vi "Main.vi"(10 "Nombre":string, 11 "Module Admin":refnum<class "Delacor_lib_QMH_Cloneable Module Admin.lvclass">) -> ()   [LabVIEW 2019, in "Inversor.lvlib"]
doc: "This template is based off of the Queued Message Handler design pattern and the Queued Message Handler project template that ships with LabVIEW.\n\nThe main difference is that the queue is private to this module and communication between modules is performed via Broadcast and Request events.\n\nRequest events are wrapped in public API methods and are handled in the Event Handling Loop (EHL) of this VI. Any module can register for Broadcast events sent by this module. The EHL generates messages based on user interface actions.\n\nThe Message Handling Loop (MHL) processes messages generated by the EHL, or by other messages. The messages are string values, so new messages can be added easily to the Message Cases case structure in the MHL. Each message cluster can also provide an optional value for Message Data, which is a variant that can be converted to whatever message-specific data is required.\n_____\nBased on DQMH Dev Tools: Project Template 7.1.0.1503."
uses:
  Inversor.lvlib
  <vilib>/Delacor/Delacor QMH/Libraries/Cloneable Module Admin_class/Delacor_lib_QMH_Cloneable Module Admin.lvclass
  C:/Program Files (x86)/National Instruments/LabVIEW 2024/vi.lib/Delacor/Delacor QMH/Libraries/Module Admin_class/Delacor_lib_QMH_Module Admin.lvclass
  Module Data--cluster.ctl
  <vilib>/Delacor/Delacor QMH/Libraries/Message Queue_class/Delacor_lib_QMH_Message Queue.lvclass/Delacor_lib_QMH_Message Queue.ctl
  <vilib>/Delacor/Delacor QMH/Libraries/Cloneable Module Admin_class/Delacor_lib_QMH_Cloneable Module Admin.lvclass/Delacor_lib_QMH_Cloneable Module Admin.ctl
  Stop Argument--cluster.ctl
  <vilib>/Delacor/Delacor QMH/Libraries/Module Admin_class/Delacor_lib_QMH_Module Admin.lvclass/Delacor_lib_QMH_Module Admin.ctl
  Request Privado Local Argument--cluster.ctl
  Request Privado Argument--cluster.ctl
  Set Voltage Argument--cluster.ctl
  Set Voltage (Reply Payload)--cluster.ctl
  Request Simple Argument--cluster.ctl
  <vilib>/Utility/miscctls.llb/LVPointTypeDef.ctl
  <vilib>/Delacor/Delacor QMH/Libraries/Message Queue_class/Delacor_lib_QMH_Enqueue Message (Single).vi
  <vilib>/Delacor/Delacor QMH/Libraries/Cloneable Module Admin_class/Delacor_lib_QMH_Get Module ID.vi
  <vilib>/Delacor/Delacor QMH/Libraries/Module Admin_class/Delacor_lib_QMH_Get External Launch.vi
  <vilib>/Delacor/Delacor QMH/Libraries/Message Queue_class/Delacor_lib_QMH_Message Queue.lvclass
panel:
  out "Active Modules (Array)":string[](array[string])
  in  "Select Module":i32(ring)=-1 caption="Select Module\nTo send Request to" items=["All"=-1]
  in  "Enviar Mensaje":bool
  in  "String":string
  out "error out":errorcluster
  out "Status":string
  in  "Simulate EHL Error":bool
  in  "Simulate MHL Error":bool
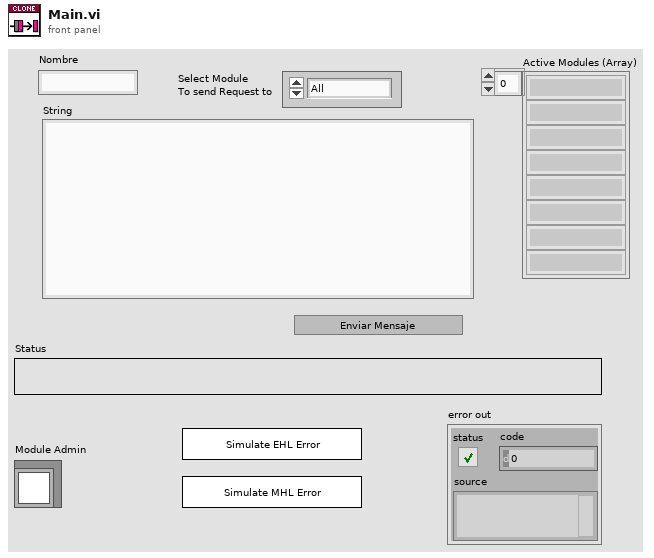
[diagram p1: front panel]
types:
  T1 = typedef "Inversor.lvlib/Broadcast Events--cluster.ctl" = cluster{"Module Did Init":refnum<user-event>, "Status Updated":refnum<user-event>, "Error Reported":refnum<user-event>, "Module Did Stop":refnum<user-event>, "Update Module Execution Status":refnum<user-event>}
  T2 = typedef "Inversor.lvlib/Request Events--cluster.ctl" = cluster{"Stop Module":refnum<user-event>, "Show Panel":refnum<user-event>, "Hide Panel":refnum<user-event>, "Show Diagram":refnum<user-event>, "Get Module Execution Status":refnum<user-event>, "Local Instance":T3, "Private.Request Privado":refnum<user-event>, "Set Voltage":refnum<user-event>, "Request Simple":refnum<user-event>}
  T3 = typedef "Inversor.lvlib/Local Instance Request Events--cluster.ctl" = cluster{"Request Privado Local":refnum<user-event>}
  T4 = typedef "Inversor.lvlib/Module Data--cluster.ctl" = cluster{"Status":string, "VISA resource name":refnum<visa-resource-name>}
  T5 = enum32{"invalid lock state", "Not Locked", "Locked (No Password)", "Password-protected"}
  T6 = typedef "Inversor.lvlib/Stop Argument--cluster.ctl" = cluster{"Module ID":i32, "Origin":string, "Exit via Stop Module Req?":bool, "Wait for Module to stop?":bool}
  T7 = typedef "Inversor.lvlib/Request Privado Local Argument--cluster.ctl" = cluster{"Module ID":i32, "Numeric":dbl}
  T8 = typedef "Inversor.lvlib/Request Privado Argument--cluster.ctl" = cluster{"Module ID":i32, "String":string}
  T9 = typedef "Inversor.lvlib/Set Voltage Argument--cluster.ctl" = cluster{"Module ID":i32, "Voltage":dbl, "Wait Notifier":refnum<notifier>, "wait for reply":bool}
  T10 = typedef "Inversor.lvlib/Request Simple Argument--cluster.ctl" = cluster{"Module ID":i32, "Numeric":dbl}
  T11 = typedef "LVPointTypeDef.ctl" = cluster{"Horizontal":i16, "Vertical":i16}
  T12 = enum32{"Invalid", "Standard", "Closed", "Hidden", "Minimized", "Maximized"}
  T13 = enum16{"Set Voltage", "Set Frecuency", "Set Speed", "Set Current"}
  T14 = typedef "Inversor.lvlib/Set Voltage (Reply Payload)--cluster.ctl" = cluster{"Module ID":i32, "Command":string, "error":errorcluster, "Response":string}
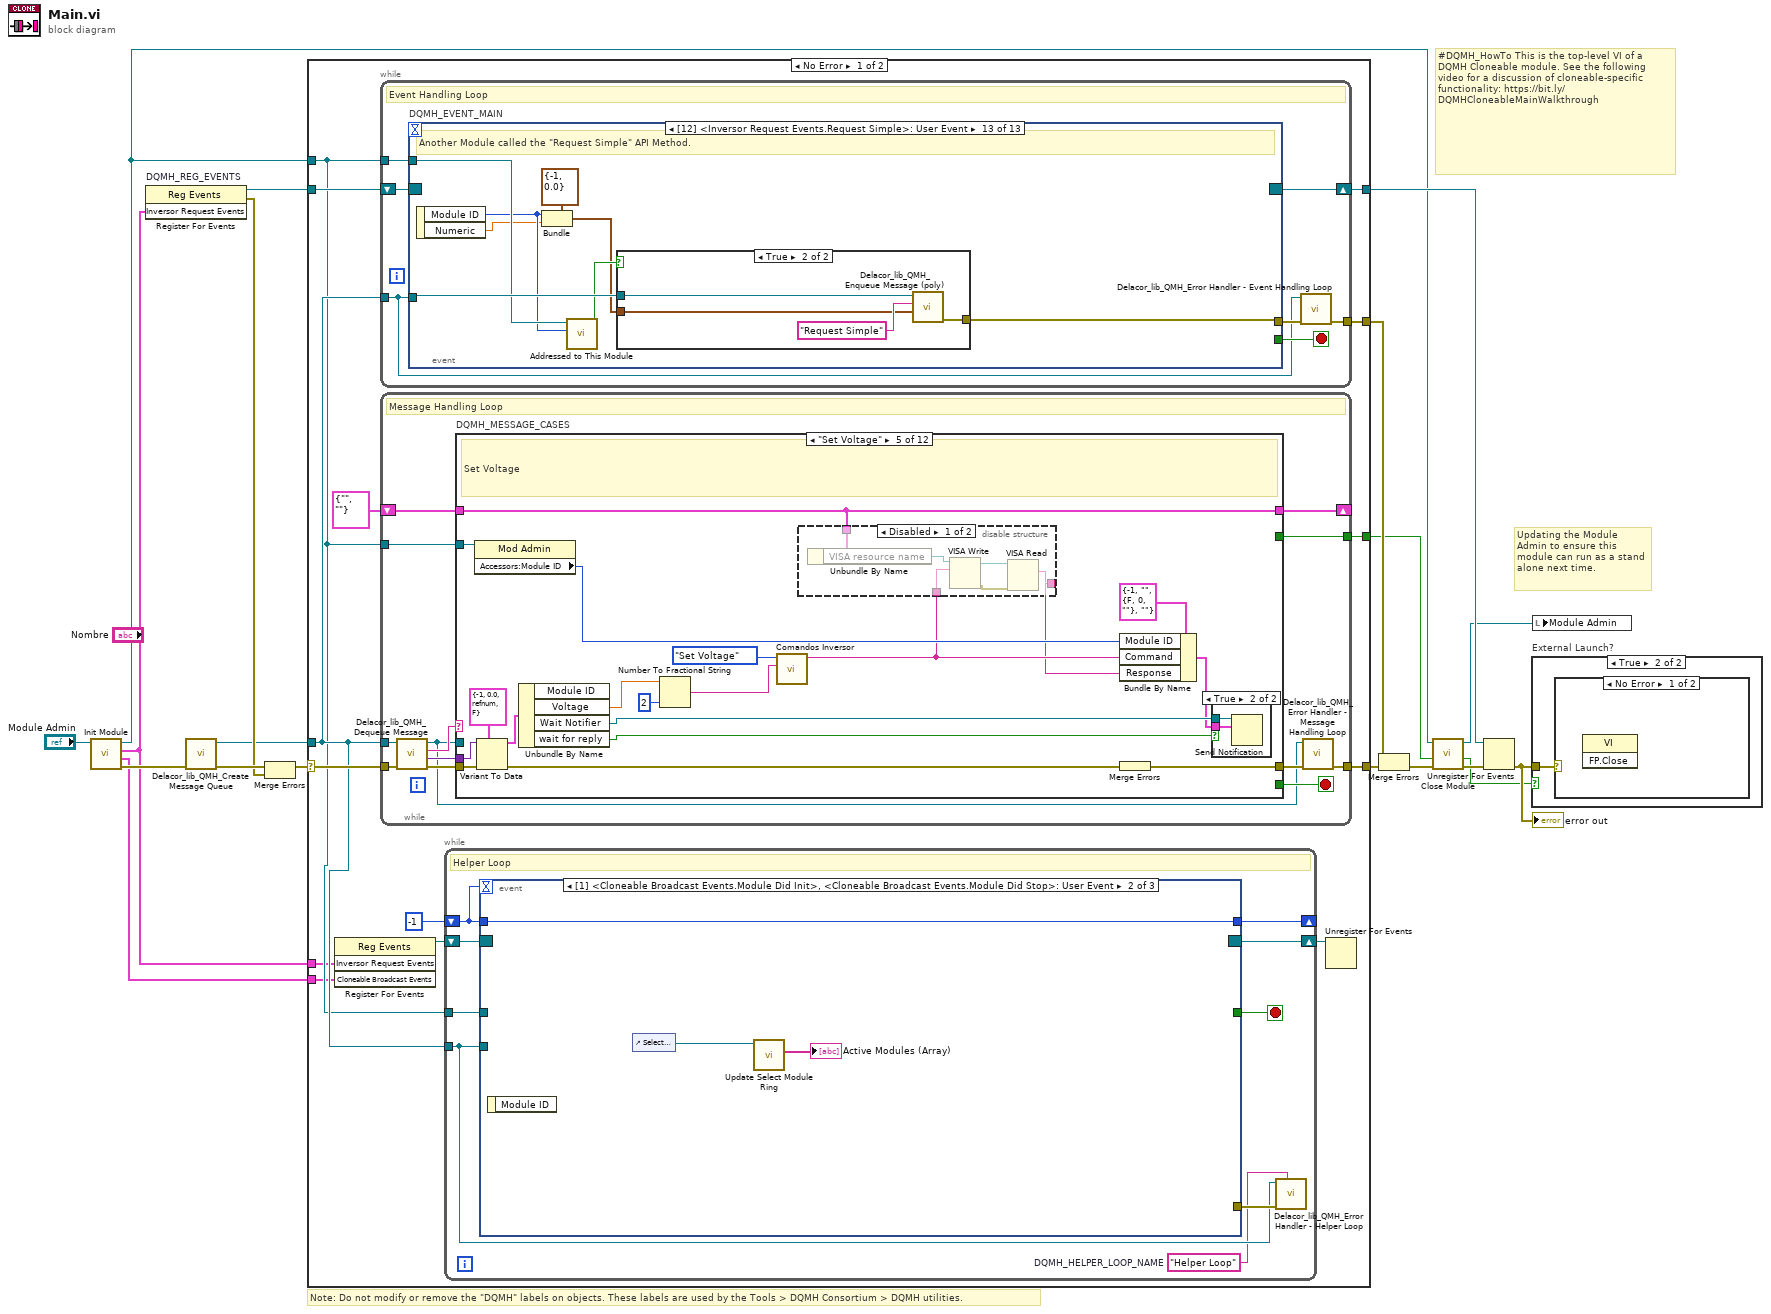
[diagram p0: block diagram]
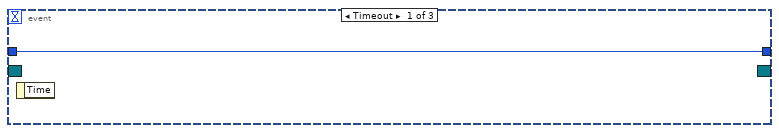
[diagram p2: hidden frame]
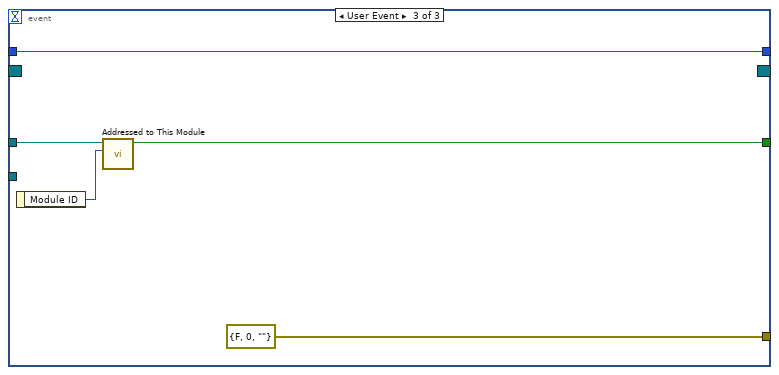
[diagram p3: hidden frame]
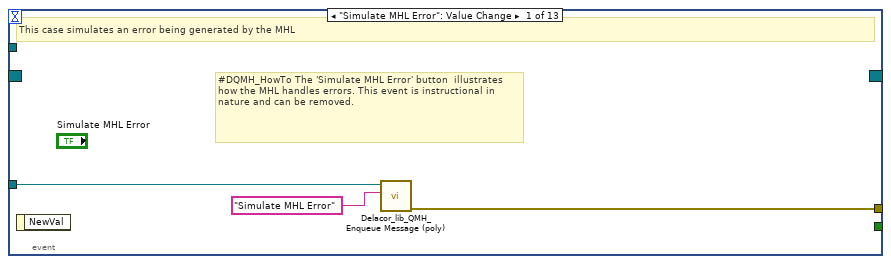
[diagram p4: hidden frame]
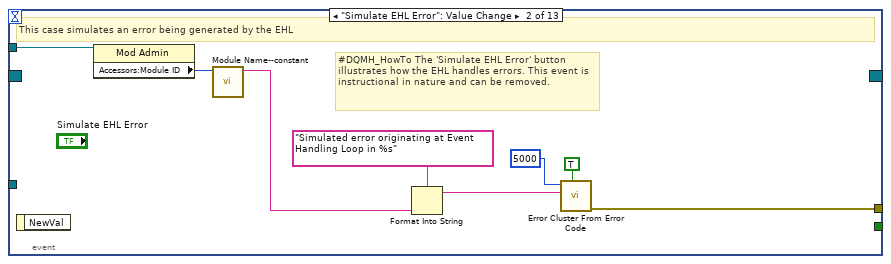
[diagram p5: hidden frame]
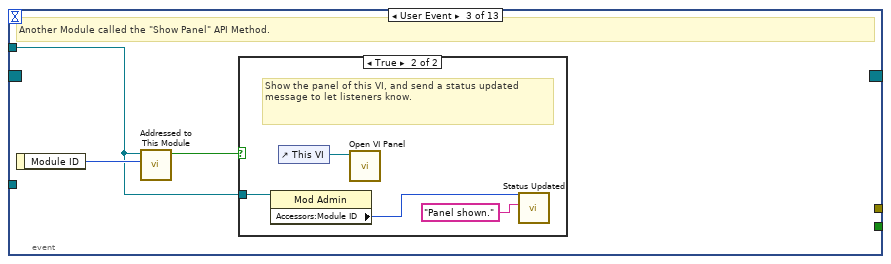
[diagram p6: hidden frame]
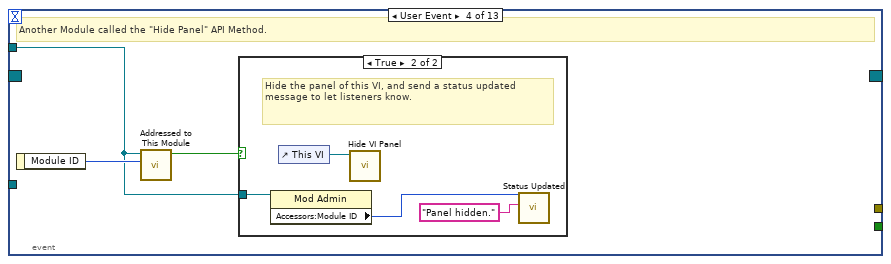
[diagram p8: hidden frame]
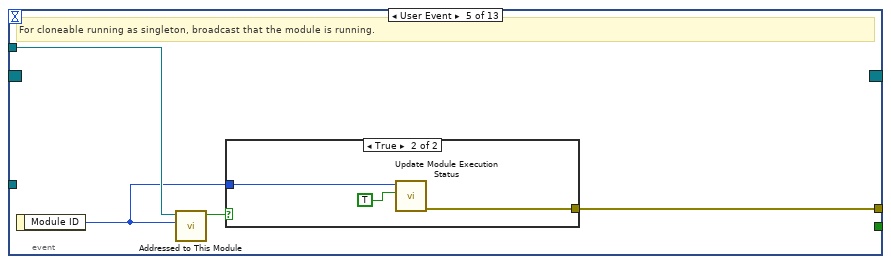
[diagram p10: hidden frame]
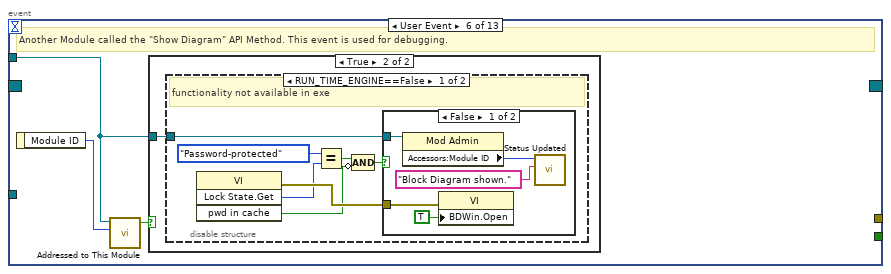
[diagram p12: hidden frame]
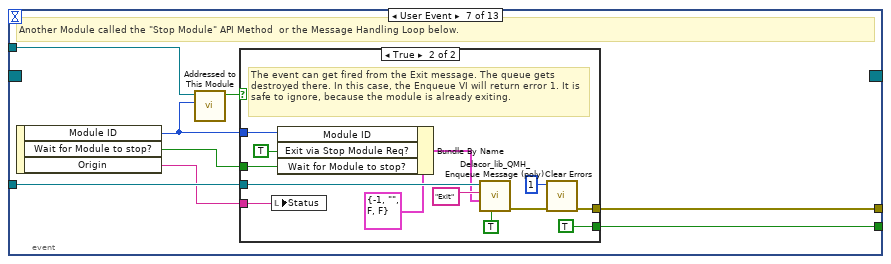
[diagram p16: hidden frame]
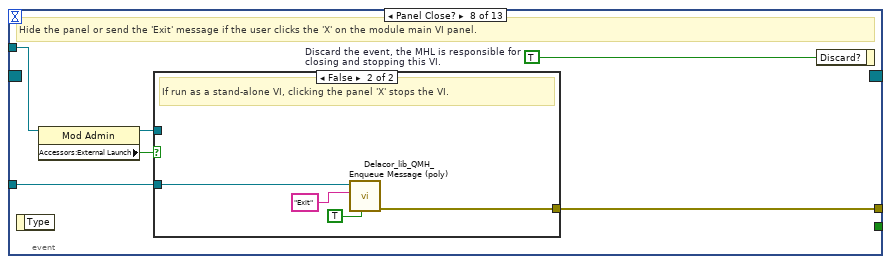
[diagram p18: hidden frame]
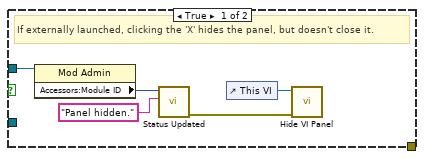
[diagram p19: hidden frame]
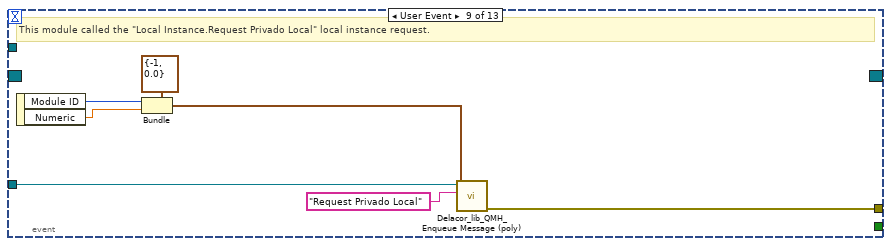
[diagram p20: hidden frame]
diagram:
  # "#DQMH_HowTo This is the top-level VI of a DQMH Cloneable module. See the following video for a discussion of cloneable-specific functionality: https://bit.ly/DQMHCloneableMainWalkthrough"
  # "Note: Do not modify or remove the \"DQMH\" labels on objects. These labels are used by the Tools > DQMH Consortium > DQMH utilities."
  # "Updating the Module Admin to ensure this module can run as a stand alone next time."
  n1 = call "Init Module.vi"("Cloneable Module Admin in"="Module Admin") -> ("error out"=w16:errorcluster, "Cloneable Broadcast Events"=w1:T1, "Inversor Request Events"=w2:T2, "Cloneable Module Admin out"=w6:refnum<class "Delacor_lib_QMH_Cloneable Module Admin.lvclass">)  [unwired: 7 in]
  n2 = register-events "DQMH_REG_EVENTS"(w2) -> (reference out=w9:refnum<event-registration>, error out=w11:errorcluster)  [unwired: 2 in]
  n3 = call <vilib>:"Delacor_lib_QMH_Create Message Queue.vi"("error in"=w16) -> ("error out"=w13:errorcluster, "Message Queue"=w8:refnum<class "Delacor_lib_QMH_Message Queue.lvclass">)  [unwired: 9 in]
  n4 = Merge Errors(w13, w11) -> (w12:errorcluster)
  n5 = case shown="No Error" w12 {
    selector: w12 -> [w31 w353]
    tunnel: [w33 w352] -> w17
    tunnel: [w30 w351] -> w10
    tunnel: w9 -> [w28 w351]
    tunnel: w8 -> [w27 w344]
    tunnel: [w32 _] -> w18
    tunnel: w6 -> [w26 w347]
    tunnel: [w25 _] -> w4
    tunnel: w2 -> [w24 _]
    tunnel: w1 -> [w20 _]
    frame No Error {
      n6 = register-events ("DQMH_HELPER_REGFOREVENTS")(w24, w20) -> (reference out=w22:refnum<event-registration>)  [unwired: 2 in, 1 out]
      n7 = while {
        tunnel: w27 -> [w52]
        shift-right: [w55] -> w30
        shift-left: w28 -> [w56]
        tunnel: [w57] -> w32
        tunnel: w26 -> [w53]
        stop <- w54 stop-if-true
        # "Event Handling Loop"
        n8 = event "DQMH_EVENT_MAIN" shown="[12] <Inversor Request Events.Request Simple>: User Event" {
          selector: w56 -> [_ _ _ _ _ _ _ _ _ _ _ _ _]
          dyn-events: [_ _ _ _ _ _ _ _ _ _ _ _ _] -> w55
          timeout: _ -> [_ _ _ _ _ _ _ _ _ _ _ _ _]
          tunnel: [_ _ _ _ _ _ w110 _ _ _ _ _ _] -> w54
          tunnel: w52 -> [w60 _ _ _ _ _ w113 w130 w149 w157 _ w173 w185]
          tunnel: [w61 w69 _ _ w87 _ w114 w133 w143 w150 _ w164 w178] -> w58
          tunnel: w53 -> [_ w68 w70 w77 w85 w91 w112 w131 _ w155 _ w171 w183]
          event "Simulate MHL Error": Value Change {
            # "#DQMH_HowTo The 'Simulate MHL Error' button  illustrates how the MHL handles errors. This event is instructional in nature and can be removed."
            # "This case simulates an error being generated by the MHL"
            n9 = event-data() -> ()  [unwired: 1 in, 1 out]
            n10 = call-poly <vilib>:"Delacor_lib_QMH_Enqueue Message (poly).vi"("Message"="Simulate MHL Error", "Message Queue in"=w60) -> ("error out"=w61:errorcluster)  [unwired: 8 in, 1 out]
          }
          event "Simulate EHL Error": Value Change {
            # "#DQMH_HowTo The 'Simulate EHL Error' button  illustrates how the EHL handles errors. This event is instructional in nature and can be removed."
            # "This case simulates an error being generated by the EHL"
            n11 = event-data() -> ()  [unwired: 1 in, 1 out]
            n12 = property on="Property Node" class="Mod Admin"(reference=w68) -> ("Accessors:Module ID"=w67:i32)  [unwired: 1 in, 2 out]
            n13 = call "Module Name--constant.vi"("Module ID"=w67) -> ("Module Name"=w62:string)  [unwired: 10 in]
            n14 = Format Into String(format string="Simulated error originating at Event Handling Loop in %s", w62) -> (resulting string=w65:string)  [unwired: 2 in, 1 out]
            n15 = call <vilib>:"Error Cluster From Error Code.vi"("show call chain? (False)"=TRUE, "error message (\"\")"=w65, "error code (0)"=5000) -> ("error out"=w69:errorcluster)  [unwired: 6 in]
          }
          event User Event {
            # "Another Module called the \"Show Panel\" API Method."
            n16 = event-data() -> ("Module ID"=w71:i32)  [unwired: 1 in]
            n17 = call "Addressed to This Module.vi"("Module ID from Argument"=w71, "Module Admin"=w70) -> ("Addressed to this instance?"=w72:bool)  [unwired: 8 in, 1 out]
            n18 = case shown="True" w72 {
              tunnel: w70 -> [_ w74]
              frame False {
              }
              frame True {
                # "Show the panel of this VI, and send a status updated message to let listeners know."
                n19 = property on="Property Node" class="Mod Admin"(reference=w74) -> ("Accessors:Module ID"=w73:i32)  [unwired: 1 in, 2 out]
                n20 = control-ref of="This VI"() -> (w76:refnum<vi>)
                n21 = call "Open VI Panel.vi"("VI"=w76) -> ()  [unwired: 10 in, 1 out]
                n22 = call "Status Updated.vi"("Status"="Panel shown." ("format string"), "Module ID"=w73) -> ()  [unwired: 9 in, 1 out]
              }
            }
          }
          event User Event {
            # "Another Module called the \"Hide Panel\" API Method."
            n23 = event-data() -> ("Module ID"=w78:i32)  [unwired: 1 in]
            n24 = call "Addressed to This Module.vi"("Module ID from Argument"=w78, "Module Admin"=w77) -> ("Addressed to this instance?"=w79:bool)  [unwired: 8 in, 1 out]
            n25 = case shown="True" w79 {
              tunnel: w77 -> [_ w81]
              frame False {
              }
              frame True {
                # "Hide the panel of this VI, and send a status updated message to let listeners know."
                n26 = property on="Property Node" class="Mod Admin"(reference=w81) -> ("Accessors:Module ID"=w80:i32)  [unwired: 1 in, 2 out]
                n27 = control-ref of="This VI"() -> (w83:refnum<vi>)
                n28 = call "Hide VI Panel.vi"("VI"=w83) -> ()  [unwired: 10 in, 1 out]
                n29 = call "Status Updated.vi"("Status"="Panel hidden." ("format string"), "Module ID"=w80) -> ()  [unwired: 9 in, 1 out]
              }
            }
          }
          event User Event {
            # "For cloneable running as singleton, broadcast that the module is running."
            n30 = event-data() -> ("Module ID"=w84:i32)  [unwired: 1 in]
            n31 = call "Addressed to This Module.vi"("Module ID from Argument"=w84, "Module Admin"=w85) -> ("Addressed to this instance?"=w86:bool)  [unwired: 8 in, 1 out]
            n32 = case shown="True" w86 {
              tunnel: [_ w90] -> w87
              tunnel: w84 -> [_ w89]
              frame False {
              }
              frame True {
                n33 = call "Update Module Execution Status.vi"("Running?"=TRUE, "Module ID"=w89) -> ("error out"=w90:errorcluster)  [unwired: 9 in]
              }
            }
          }
          event User Event {
            # "Another Module called the \"Show Diagram\" API Method. This event is used for debugging."
            n34 = event-data() -> ("Module ID"=w92:i32)  [unwired: 1 in]
            n35 = call "Addressed to This Module.vi"("Module ID from Argument"=w92, "Module Admin"=w91) -> ("Addressed to this instance?"=w93:bool)  [unwired: 8 in, 1 out]
            n36 = case shown="True" w93 {
              tunnel: w91 -> [_ w94]
              frame False {
              }
              frame True {
                n37 = disable-structure shown="RUN_TIME_ENGINE==False" {
                  disable-tunnel: w94 -> [w95 _]
                  frame condition #0 (active) {
                    # "functionality not available in exe"
                    n38 = invoke on="Invoke Node" class="VI" method="Lock State.Get"() -> (error out=w101:errorcluster, "Get Lock State"=w100:T5, "pwd in cache"=w97:bool)  [unwired: 4 in, 1 out]
                    n39 = Equal?(x=T5."Password-protected", y=w100) -> (x = y?=w98:bool)
                    n40 = Compound Arithmetic op=AND(w98, invert w97) -> (w96:bool)
                    n41 = case shown="False" w96 {
                      tunnel: w101 -> [w106 _]
                      tunnel: w95 -> [w103 _]
                      frame False {
                        n42 = property on="Property Node" class="Mod Admin"(reference=w103) -> ("Accessors:Module ID"=w102:i32)  [unwired: 1 in, 2 out]
                        n43 = property on="Property Node" class="VI"(error in=w106, "BDWin.Open"=TRUE ("Block Diagram Window:Open")) -> ()  [unwired: 1 in, 2 out]
                        n44 = call "Status Updated.vi"("Status"="Block Diagram shown." ("format string"), "Module ID"=w102) -> ()  [unwired: 9 in, 1 out]
                      }
                      frame True {
                        # "Password-protected VI, and the password is not in the cache. Do not show the diagram."
                      }
                    }
                  }
                  frame condition #1 {
                  }
                }
              }
            }
          }
          event User Event {
            # "Another Module called the \"Stop Module\" API Method  or the Message Handling Loop below."
            n45 = event-data() -> ("Module ID"=w108:i32, "Wait for Module to stop?"=w109:bool, "Origin"=w107:string)  [unwired: 1 in]
            n46 = call "Addressed to This Module.vi"("Module ID from Argument"=w108, "Module Admin"=w112) -> ("Addressed to this instance?"=w111:bool)  [unwired: 8 in, 1 out]
            n47 = case shown="True" w111 {
              tunnel: [_ w126] -> w114
              tunnel: w113 -> [_ w122]
              tunnel: [_ TRUE] -> w110
              tunnel: w109 -> [_ w117]
              tunnel: w108 -> [_ w119]
              tunnel: w107 -> [_ w115]
              frame False {
              }
              frame True {
                # "The event can get fired from the Exit message. The queue gets destroyed there. In this case, the Enqueue VI will return error 1. It is safe to ignore, because the module is already exiting."
                n48 = local write "Status"(w115) -> ()
                n49 = Bundle By Name(cluster=T6 {"Module ID"=-1, "Origin"="", "Exit via Stop Module Req?"=FALSE, "Wait for Module to stop?"=FALSE} ("Stop Argument"), "Module ID"=w119, "Exit via Stop Module Req?"=TRUE, "Wait for Module to stop?"=w117) -> (w116:T6)
                n50 = call-poly <vilib>:"Delacor_lib_QMH_Enqueue Message (poly).vi"("Priority Message? (F)"=TRUE, "Message Data"=w116, "Message"="Exit", "Message Queue in"=w122) -> ("error out"=w127:errorcluster)  [unwired: 6 in, 1 out]
                n51 = call <vilib>:"Clear Errors.vi"("error in (no error)"=w127, "specific error code to clear (0: all)"=1) -> ("error out"=w126:errorcluster)  [unwired: 4 in, 1 out]
              }
            }
          }
          event Panel Close? {
            w132 = TRUE  # Discard the event, the MHL is responsible for closing and stopping this VI.
            # "Hide the panel or send the 'Exit' message if the user clicks the 'X' on the module main VI panel."
            n52 = event-data() -> ()  [unwired: 1 in, 1 out]
            n53 = property on="Property Node" class="Mod Admin"(reference=w131) -> (reference out=w128:refnum<class "Delacor_lib_QMH_Cloneable Module Admin.lvclass">, "Accessors:External Launch"=w129:bool)  [unwired: 1 in, 1 out]
            n54 = case shown="False" w129 {
              tunnel: w130 -> [_ w141]
              tunnel: [_ w142] -> w133
              tunnel: w128 -> [w136 _]
              frame True {
                # "If externally launched, clicking the 'X' hides the panel, but doesn't close it."
                n55 = property on="Property Node" class="Mod Admin"(reference=w136) -> ("Accessors:Module ID"=w135:i32)  [unwired: 1 in, 2 out]
                n56 = call "Status Updated.vi"("Status"="Panel hidden." ("format string"), "Module ID"=w135) -> ("error out"=w134:errorcluster)  [unwired: 9 in]
                n57 = control-ref of="This VI"() -> (w138:refnum<vi>)
                n58 = call "Hide VI Panel.vi"("error in"=w134, "VI"=w138) -> ()  [unwired: 9 in, 1 out]
              }
              frame False {
                # "If run as a stand-alone VI, clicking the panel 'X' stops the VI."
                n59 = call-poly <vilib>:"Delacor_lib_QMH_Enqueue Message (poly).vi"("Priority Message? (F)"=TRUE, "Message"="Exit", "Message Queue in"=w141) -> ("error out"=w142:errorcluster)  [unwired: 7 in, 1 out]
              }
            }
            n60 = event-data ("Event Filter Node")("Discard?"=w132) -> ()  [unwired: 1 in, 1 out]
          }
          event User Event {
            # "This module called the \"Local Instance.Request Privado Local\" local instance request."
            n61 = event-data() -> ("Module ID"=w145:i32, "Numeric"=w144:dbl)  [unwired: 1 in]
            n62 = Bundle(cluster=T7 {"Module ID"=-1, "Numeric"=0.0} ("Request Privado Local Argument"), "Module ID"=w145, "Numeric"=w144) -> (w146:T7)
            n63 = call-poly <vilib>:"Delacor_lib_QMH_Enqueue Message (poly).vi"("Message Data"=w146, "Message"="Request Privado Local", "Message Queue in"=w149) -> ("error out"=w143:errorcluster)  [unwired: 7 in, 1 out]
          }
          event User Event {
            # "This module called the \"Private.Request Privado\" private request."
            n64 = event-data() -> ("Module ID"=w152:i32, "String"=w151:string)  [unwired: 1 in]
            n65 = Bundle(cluster=T8 {"Module ID"=-1, "String"=""} ("Request Privado Argument"), "Module ID"=w152, "String"=w151) -> (w153:T8)
            n66 = call "Addressed to This Module.vi"("Module ID from Argument"=w152, "Module Admin"=w155) -> ("Addressed to this instance?"=w156:bool)  [unwired: 8 in, 1 out]
            n67 = case shown="True" w156 {
              tunnel: w157 -> [_ w161]
              tunnel: w153 -> [_ w159]
              tunnel: [_ w158] -> w150
              frame False {
              }
              frame True {
                n68 = call-poly <vilib>:"Delacor_lib_QMH_Enqueue Message (poly).vi"("Message Data"=w159, "Message"="Request Privado", "Message Queue in"=w161) -> ("error out"=w158:errorcluster)  [unwired: 7 in, 1 out]
              }
            }
          }
          event "Enviar Mensaje": Value Change {
            n69 = event-data() -> ()  [unwired: 1 in, 1 out]
            n70 = call "Request Privado.vi"("String"="String", "Module ID"="Select Module") -> ()  [unwired: 9 in, 1 out]
          }
          event User Event {
            # "Another Module called the \"Set Voltage\" API Method."
            n71 = event-data() -> ("Module ID"=w168:i32, "Voltage"=w167:dbl, "Wait Notifier"=w166:refnum<notifier>, "wait for reply"=w165:bool)  [unwired: 1 in]
            n72 = Bundle(cluster=T9 {"Module ID"=-1, "Voltage"=0.0, "Wait Notifier"=refnum, "wait for reply"=FALSE} ("Set Voltage Argument"), "Module ID"=w168, "Voltage"=w167, "Wait Notifier"=w166, "wait for reply"=w165) -> (w169:T9)
            n73 = call "Addressed to This Module.vi"("Module ID from Argument"=w168, "Module Admin"=w171) -> ("Addressed to this instance?"=w172:bool)  [unwired: 8 in, 1 out]
            n74 = case shown="True" w172 {
              tunnel: w173 -> [_ w177]
              tunnel: w169 -> [_ w175]
              tunnel: [_ w174] -> w164
              frame False {
              }
              frame True {
                n75 = call-poly <vilib>:"Delacor_lib_QMH_Enqueue Message (poly).vi"("Message Data"=w175, "Message"="Set Voltage", "Message Queue in"=w177) -> ("error out"=w174:errorcluster)  [unwired: 7 in, 1 out]
              }
            }
          }
          event User Event {
            # "Another Module called the \"Request Simple\" API Method."
            n76 = event-data() -> ("Module ID"=w180:i32, "Numeric"=w179:dbl)  [unwired: 1 in]
            n77 = Bundle(cluster=T10 {"Module ID"=-1, "Numeric"=0.0} ("Request Simple Argument"), "Module ID"=w180, "Numeric"=w179) -> (w181:T10)
            n78 = call "Addressed to This Module.vi"("Module ID from Argument"=w180, "Module Admin"=w183) -> ("Addressed to this instance?"=w184:bool)  [unwired: 8 in, 1 out]
            n79 = case shown="True" w184 {
              tunnel: w185 -> [_ w189]
              tunnel: w181 -> [_ w187]
              tunnel: [_ w186] -> w178
              frame False {
              }
              frame True {
                n80 = call-poly <vilib>:"Delacor_lib_QMH_Enqueue Message (poly).vi"("Message Data"=w187, "Message"="Request Simple", "Message Queue in"=w189) -> ("error out"=w186:errorcluster)  [unwired: 7 in, 1 out]
              }
            }
          }
        }
        n81 = call-dynamic "Delacor_lib_QMH_Error Handler - Event Handling Loop.vi"("error in"=w58, "Message Queue in"=w52) -> ("dup error in"=w57:errorcluster)  [unwired: 8 in, 1 out]
      }
      n82 = while {
        tunnel: w27 -> [w190]
        shift-right: [w197] -> _
        shift-left: T4 {"Status"="", "VISA resource name"=""} ("Data Cluster") -> [w198]
        tunnel: w31 -> [w201]
        tunnel: [w199] -> w33
        tunnel: w26 -> [w192]
        tunnel: [w191] -> w25
        stop <- w196 stop-if-true
        # "Message Handling Loop"
        n83 = call-dynamic "Delacor_lib_QMH_Dequeue Message.vi"("error in"=w201, "Message Queue in"=w190) -> ("error out"=w200:errorcluster, "Message Data"=w194:variant, "Message"=w195:string, "Message Queue out"=w193:refnum<class "Delacor_lib_QMH_Message Queue.lvclass">)  [unwired: 6 in]
        n84 = case "DQMH_MESSAGE_CASES" shown="\"Set Voltage\"" w195 {
          selector: w195 -> [_ _ _ _ _ _ _ _ _ _ _ w333]
          tunnel: w193 -> [_ _ _ _ _ _ _ _ w288 _ w325 _]
          tunnel: w200 -> [w222 w226 w232 w243 w262 w280 w283 w285 w297 w314 w331 w342]
          tunnel: [w220 w226 w230 w241 w253 w278 w282 w285 w293 w313 w326 w343] -> w202
          tunnel: w198 -> [w213 w225 w231 w242 w246 w279 w281 w284 w292 w311 w324 w340]
          tunnel: [w212 w225 w231 w242 w246 w279 w281 w284 w292 w311 w324 w340] -> w197
          tunnel: [_ _ _ _ _ _ _ _ _ _ w323 _] -> w196
          tunnel: w194 -> [_ _ w229 w240 w260 w277 _ _ w291 _ w321 _]
          tunnel: w192 -> [w208 _ _ w237 w251 w274 _ _ w290 w309 w316 w339]
          tunnel: [_ _ _ _ _ _ _ _ _ _ w319 _] -> w191
          frame "Initialize" {
            w205 = "Initial Message" ("Initial Message")
            # "#DQMH_CodeNeeded - Initialize the appearance of the front panel."
            # "#DQMH_CodeNeeded - Initialize your state data here."
            # "Initialize - Any operation that needs to be done before the module can receive messages. Synchronize Caller Events.vi will inform Start Module.vi that the module has launched and is ready to receive messages. Module Did Init.vi will broadcast that the module initialized."
            n85 = call "Synchronize Caller Events.vi"("error in"=w222, "Module Admin"=w208) -> ("error out"=w221:errorcluster, "Module Admin out"=w207:refnum<class "Delacor_lib_QMH_Cloneable Module Admin.lvclass">)  [unwired: 8 in]
            n86 = property on="Property Node" class="Mod Admin"(reference=w207) -> ("Accessors:Module ID"=w204:i32, "Accessors:External Launch"=w209:bool)  [unwired: 1 in, 2 out]
            n87 = call "Module Name--constant.vi"("Module ID"=w204) -> ("Module Name"=w217:string)  [unwired: 10 in]
            n88 = property on="Property Node" class="VI"("Front Panel.Title"=w217) -> (reference out=w219:refnum<vi>, error out=w224:errorcluster)  [unwired: 2 in]
            n89 = Select(t=T12."Hidden" ("State"), s=w209, f=T12."Standard" ("State")) -> (s? t:f=w214:T12)
            n90 = invoke on="Invoke Node" class="VI" method="FP.Open"(reference=w219, error in=w224, "State"=w214) -> (reference out=w218:refnum<vi>, error out=w223:errorcluster)  [unwired: 2 in, 3 out]
            n91 = Bundle By Name(cluster=w213, "Status"=w205) -> (w212:T4)
            n92 = invoke on="Invoke Node" class="VI" method="FP.Center"(reference=w218, error in=w223) -> ()  [unwired: 1 in, 3 out]
            n93 = property on="Pane" class="Pane"("Origin"=T11 {"Horizontal"=0, "Vertical"=0}) -> ()  [unwired: 2 in, 2 out]
            n94 = call "Request Privado Local.vi"("Numeric"=123.0, "Module ID"=w204) -> ()  [unwired: 9 in, 1 out]
            n95 = call "Module Name--constant.vi"("Module ID"=w204) -> ("Module Name"=w210:string)  [unwired: 10 in]
            n96 = call "Module Did Init.vi"("error in"=w221, "Initialized?"=TRUE, "Origin"=w210, "Module ID"=w204) -> ("error out"=w220:errorcluster)  [unwired: 7 in]
            "Status" <- w205
          }
          frame "---Module Specific---" {
            # "Separator -- The following cases handle messages specific to this Module."
          }
          frame "Request Privado Local" {
            n97 = Variant To Data(error in=w232, type=T7 {"Module ID"=-1, "Numeric"=0.0} ("Request Privado Local Argument"), Variant=w229) -> (data=w227:T7, error out=w230:errorcluster)
            n98 = Unbundle By Name(w227) -> ()  [unwired: 2 out]
          }
          frame "Request Privado" {
            n99 = Variant To Data(error in=w243, type=T8 {"Module ID"=-1, "String"=""} ("Request Privado Argument"), Variant=w240) -> (data=w238:T8, error out=w241:errorcluster)
            n100 = property class="Mod Admin"(reference=w237) -> ("Accessors:Module ID"=w236:i32)  [unwired: 1 in, 2 out]
            n101 = Unbundle By Name(w238) -> ("String"=w235:string)
            n102 = Format Into String(format string="Module ID:%d Mensaje recibido: %s", w236, w235) -> (resulting string=w234:string)  [unwired: 2 in, 1 out]
            n103 = One Button Dialog(message=w234) -> ()  [unwired: 1 in, 1 out]
          }
          frame "Set Voltage" {
            # "Set Voltage"
            n104 = property class="Mod Admin"(reference=w251) -> ("Accessors:Module ID"=w252:i32)  [unwired: 1 in, 2 out]
            n105 = Variant To Data(error in=w262, type=T9 {"Module ID"=-1, "Voltage"=0.0, "Wait Notifier"=refnum, "wait for reply"=FALSE} ("Set Voltage Argument"), Variant=w260) -> (data=w258:T9, error out=w261:errorcluster)
            n106 = Unbundle By Name(w258) -> ("Voltage"=w249:dbl, "Wait Notifier"=w257:refnum<notifier>, "wait for reply"=w256:bool)  [unwired: 1 out]
            n107 = Number To Fractional String(number=w249, precision (6)=i16 2) -> (F-format string=w248:string)  [unwired: 2 in]
            n108 = call "Comandos Inversor.vi"("Argument"=w248, "Command"=T13."Set Voltage") -> ("Command"=w245:string)  [unwired: 9 in]
            n109 = disable-structure shown="Disabled" {
              disable-tunnel: w246 -> [w268 _]
              disable-tunnel: w245 -> [w266 _]
              disable-tunnel: [w263 _] -> w244
              frame Disabled {
                n110 = Unbundle By Name(w268) -> ("VISA resource name"=w267:refnum<visa-resource-name>)
                n111 = VISA Write(VISA resource name=w267, write buffer=w266) -> (VISA resource name out=w265:refnum<visa-resource-name>, error out=w264:errorcluster)  [unwired: 1 in, 1 out]
                n112 = VISA Read(VISA resource name=w265, error in (no error)=w264) -> (read buffer=w263:string)  [unwired: 1 in, 3 out]
              }
              frame Enabled {
              }
            }
            n113 = Bundle By Name(cluster=T14 {"Module ID"=-1, "Command"="", "error"={"status"=FALSE, "code"=0, "source"=""}, "Response"=""} ("Set Voltage (Reply Payload)"), "Module ID"=w252, "Command"=w245, "Response"=w244) -> (w255:T14)
            n114 = Merge Errors(w261) -> (w253:errorcluster)
            n115 = case "DQMH_FIRE_NOTIFIER" shown="True" w256 {
              tunnel: w257 -> [_ w270]
              tunnel: w255 -> [_ w269]
              frame False {
              }
              frame True {
                n116 = Send Notification(notification=w269, notifier=w270) -> ()  [unwired: 1 in, 2 out]
              }
            }
          }
          frame "Request Simple" {
            n117 = Variant To Data(error in=w280, type=T10 {"Module ID"=-1, "Numeric"=0.0} ("Request Simple Argument"), Variant=w277) -> (data=w275:T10, error out=w278:errorcluster)
            n118 = Unbundle By Name(w275) -> ("Numeric"=w272:dbl)  [unwired: 1 out]
            n119 = property class="Mod Admin"(reference=w274) -> ("Accessors:Module ID"=w273:i32)  [unwired: 1 in, 2 out]
            n120 = Format Into String(w272) -> (resulting string=w271:string)  [unwired: 3 in, 1 out]
            n121 = call "Status Updated.vi"("Status"=w271, "Module ID"=w273) -> ()  [unwired: 9 in, 1 out]
          }
          frame "---Copy This Frame---" {
            # "Duplicate this frame when creating new messages.  Change this comment in the duplicated frame to describe this message."
            n122 = Merge Errors(w283) -> (w282:errorcluster)
          }
          frame "---Exit and Error Handling---" {
            # "Separator - the following cases handle errors and exit messages."
          }
          frame "Error" {
            # "#DQMH_CodeRecommended - If the module is running in standalone mode (External Launch = FALSE), this code will pop up an error dialog and call the 'Exit' message if an error occurs. Add more fine-grained error management here."
            # "Error - Check the error message data and respond accordingly. This message is sent by the \"Error Handler\" VIs at the end of each loop in this application."
            n123 = property on="Property Node" class="Mod Admin"(reference=w290) -> ("Accessors:External Launch"=w289:bool, "Accessors:Module ID"=w287:i32)  [unwired: 1 in, 2 out]
            n124 = Variant To Data(error in=w297, type=errorcluster {"status"=FALSE, "code"=0, "source"=""} ("error constant"), Variant=w291) -> (data=w286:errorcluster, error out=w295:errorcluster)
            n125 = local write "error out"(w286) -> ()
            n126 = call "Error Reported.vi"("Error"=w286, "Module ID"=w287) -> ()  [unwired: 9 in, 1 out]
            n127 = case shown="False" w289 {
              tunnel: [w302 _] -> w294
              tunnel: w288 -> [w300 _]
              tunnel: w286 -> [w301 _]
              frame False {
                n128 = disable-structure shown="Default" {
                  disable-tunnel: w301 -> [w303 _]
                  frame condition #0 (active) {
                    # "If the module is running standalone, then pop up an error dialog and call the \"Exit\" message."
                    n129 = call <vilib>:"Simple Error Handler.vi"("error in (no error)"=w303) -> ()  [unwired: 4 in, 5 out]
                  }
                  frame condition #1 {
                    # "To prevent the Simple Error Handler VI from being loaded (e.g. when deploying to a Real-Time target), add the Conditional Disable Symbol \"DQMH_Disable_SEH\" to your project and set it to TRUE."
                  }
                }
                n130 = call-poly <vilib>:"Delacor_lib_QMH_Enqueue Message (poly).vi"("Priority Message? (F)"=TRUE, "Message"="Exit", "Message Queue in"=w300) -> ("error out"=w302:errorcluster)  [unwired: 7 in, 1 out]
              }
              frame True {
                # "If the module was launched externally, calling the Error Reported broadcast VI is the only action performed by the \"Error\" message. The module's caller can then process the error appropriately."
              }
            }
            n131 = Merge Errors(w295, w294) -> (w293:errorcluster)
          }
          frame "Simulate MHL Error" {
            # "#DQMH_HowTo The 'Simulate MHL Error' button  illustrates how the MHL handles errors. This event is instructional in nature and can be removed."
            # "Simulate an error occurring at the MHL"
            n132 = property on="Property Node" class="Mod Admin"(reference=w309) -> ("Accessors:Module ID"=w310:i32)  [unwired: 1 in, 2 out]
            n133 = call "Module Name--constant.vi"("Module ID"=w310) -> ("Module Name"=w305:string)  [unwired: 10 in]
            n134 = Format Into String(format string="Simulated error originating at Message Handling Loop in %s", w305) -> (resulting string=w306:string)  [unwired: 2 in, 1 out]
            n135 = call <vilib>:"Error Cluster From Error Code.vi"("show call chain? (False)"=TRUE, "error message (\"\")"=w306, "error code (0)"=5001) -> ("error out"=w312:errorcluster)  [unwired: 6 in]
            n136 = Merge Errors(w314, w312) -> (w313:errorcluster)
          }
          frame "Exit" {
            w322 = 91  # 91: not all Exit messages will have an argument
            w323 = TRUE  # Stop the VI
            # "Release the message queue reference"
            # "#DQMH_CodeNeeded - Add any required cleanup code here."
            # "Exit - Exit the application."
            n137 = Variant To Data(error in=w331, type=T6 {"Module ID"=-1, "Origin"="", "Exit via Stop Module Req?"=FALSE, "Wait for Module to stop?"=FALSE} ("Stop Argument"), Variant=w321) -> (data=w318:T6, error out=w327:errorcluster)
            n138 = call <vilib>:"Clear Errors.vi"("error in (no error)"=w327, "specific error code to clear (0: all)"=w322) -> ("error out"=w330:errorcluster)  [unwired: 4 in, 1 out]
            n139 = property on="Property Node" class="Mod Admin"(reference=w316) -> ("Accessors:Module ID"=w315:i32)  [unwired: 1 in, 2 out]
            n140 = control-ref of="This VI"() -> (w317:refnum<vi>)
            n141 = call-dynamic "Delacor_lib_QMH_Release Message Queue.vi"("error in"=w330, "Message Queue"=w325) -> ("error out"=w329:errorcluster)  [unwired: 9 in]
            n142 = call "Handle Exit.vi"("Stop Argument"=w318, "Module Admin in"=w316, "VI reference"=w317) -> ("error out"=w328:errorcluster, "Wait for Stop?"=w319:bool)  [unwired: 7 in]
            n143 = Merge Errors(w329, w328) -> (w326:errorcluster)
            n144 = call "Error Reported.vi"("Error"=w326, "Module ID"=w315) -> ()  [unwired: 9 in, 1 out]
          }
          frame Default {
            # "'Default' case only runs if there is a message that isn't defined in any of the other cases.  Output a programming error."
            n145 = property on="Property Node" class="Mod Admin"(reference=w339) -> ("Accessors:Module ID"=w338:i32)  [unwired: 1 in, 2 out]
            n146 = call "Module Name--constant.vi"("Module ID"=w338) -> ("Module Name"=w332:string)  [unwired: 10 in]
            n147 = Format Into String(format string="The invalid message string \"%s\" was received in the Message Handling Loop for module \"%s\".", w333, w332) -> (resulting string=w335:string)  [unwired: 2 in, 1 out]
            n148 = call <vilib>:"Error Cluster From Error Code.vi"("show call chain? (False)"=TRUE, "error message (\"\")"=w335, "error code (0)"=1) -> ("error out"=w341:errorcluster)  [unwired: 6 in]
            n149 = Merge Errors(w342, w341) -> (w343:errorcluster)
          }
        }
        n150 = call-dynamic "Delacor_lib_QMH_Error Handler - Message Handling Loop.vi"("error in"=w202, "Message Queue in"=w193) -> ("dup error in"=w199:errorcluster)  [unwired: 8 in, 1 out]
      }
      n151 = while "DQMH_HELPER_LOOP" {
        shift-right: [w42] -> _
        shift-left: -1 -> [w41]
        shift-right: [w39] -> w23
        shift-left: w22 -> [w40]
        tunnel: w27 -> [w36]
        tunnel: w26 -> [w34]
        stop <- w38 stop-if-true
        w35 = "Helper Loop"  # DQMH_HELPER_LOOP_NAME
        # "Helper Loop"
        n152 = event "DQMH_HELPER_EVENT_STRUCTURE" shown="[1] <Cloneable Broadcast Events.Module Did Init>, <Cloneable Broadcast Events.Module Did Stop>: User Event" {
          selector: w40 -> [_ _ _]
          dyn-events: [_ _ _] -> w39
          timeout: w41 -> [_ _ _]
          tunnel: w41 -> [w43 w46 w51]
          tunnel: [w43 w46 w51] -> w42
          tunnel: [_ _ w48] -> w38
          tunnel: [_ _ errorcluster {"status"=FALSE, "code"=0, "source"=""} ("error constant")] -> w37
          tunnel: w36 -> [_ _ _]
          tunnel: w34 -> [_ _ w49]
          event Timeout {
            n153 = event-data() -> ()  [unwired: 1 in, 1 out]
          }
          event User Event {
            n154 = event-data() -> ()  [unwired: 1 in, 1 out]
            n155 = control-ref of="Select Module"() -> (w45:refnum<vi>)
            n156 = call "Update Select Module Ring.vi"("Select Module Ring Ref"=w45) -> ("Active Modules (Array)"=→"Active Modules (Array)":string[])  [unwired: 8 in, 2 out]
          }
          event User Event {
            n157 = event-data() -> ("Module ID"=w47:i32)  [unwired: 1 in]
            n158 = call "Addressed to This Module.vi"("Module ID from Argument"=w47, "Module Admin"=w49) -> ("Addressed to this instance?"=w48:bool)  [unwired: 8 in, 1 out]
          }
        }
        n159 = call-dynamic "Delacor_lib_QMH_Error Handler - Helper Loop.vi"("Error Debug"=w35, "error in"=w37, "Message Queue in"=w36) -> ()  [unwired: 7 in, 2 out]
      }
      n160 = Unregister For Events(event registration refnum=w23) -> ()  [unwired: 1 in, 1 out]
    }
    frame Error {
      n161 = call "Synchronize Caller Events.vi"("Module Admin"=w347) -> ("Module Admin out"=w346:refnum<class "Delacor_lib_QMH_Cloneable Module Admin.lvclass">)  [unwired: 9 in, 1 out]
      n162 = property on="Property Node" class="Mod Admin"(reference=w346) -> ("Accessors:Module ID"=w345:i32)  [unwired: 1 in, 2 out]
      n163 = call-dynamic "Delacor_lib_QMH_Release Message Queue.vi"("error in"=w353, "Message Queue"=w344) -> ("error out"=w352:errorcluster)  [unwired: 9 in]
      n164 = call "Module Name--constant.vi"("Module ID"=w345) -> ("Module Name"=w350:string)  [unwired: 10 in]
      n165 = Format Into String(format string="An error occurred during initialization. %s is no longer running.", w350) -> (resulting string=w348:string)  [unwired: 2 in, 1 out]
      n166 = call "Error Reported.vi"("Additional Information"=w348, "Error"=w352, "Module ID"=w345) -> ()  [unwired: 8 in, 1 out]
    }
  }
  n167 = Merge Errors(w18, w17) -> (w19:errorcluster)
  n168 = call "Close Module.vi"("error in"=w19, "Wait for stop?"=w4, "Module Admin in"=w6) -> ("error out"=w15:errorcluster, "External Launch"=w3:bool, "Module Admin out"=w5:refnum<class "Delacor_lib_QMH_Cloneable Module Admin.lvclass">)  [unwired: 6 in]
  n169 = Unregister For Events(event registration refnum=w10, error in=w15) -> (error out=w14:errorcluster)
  "error out" <- w14
  n170 = case "External Launch?" shown="True" w3 {
    tunnel: w14 -> [_ w354]
    frame False {
    }
    frame True {
      n171 = case shown="No Error" w354 {
        frame No Error {
          n172 = invoke class="VI" method="FP.Close"() -> ()  [unwired: 3 in, 3 out]
        }
        frame Error {
          n173 = disable-structure shown="Default" {
            frame condition #0 (active) {
              n174 = invoke class="VI" method="FP.Open"("Activate"=TRUE ("Activate?")) -> ()  [unwired: 4 in, 5 out]
            }
            frame condition #1 {
              # "Don't show panel on error if running inside a built EXE."
            }
          }
        }
      }
    }
  }
  n175 = local write "Module Admin"(w5) -> ()
